vi "Restore Connection.vi"(8 "error in (no error)":errorcluster, 11 "Spectrum Recorder too in":refnum<class "Spectrum Recorder too.lvclass">) -> (0 "error out":errorcluster, 1 "Attempts":i32, 2 "Time elapsed, ms":u32, 3 "Spectrum Recorder too out":refnum<class "Spectrum Recorder too.lvclass">)   [LabVIEW 2020, in "Spectrum Recorder too.lvclass"]
uses:
  Spectrum Recorder too.lvclass
  <vilib>/Utility/error.llb/Error Cluster From Error Code.vi
  <vilib>/ErrorRing/Error Ring.xnode
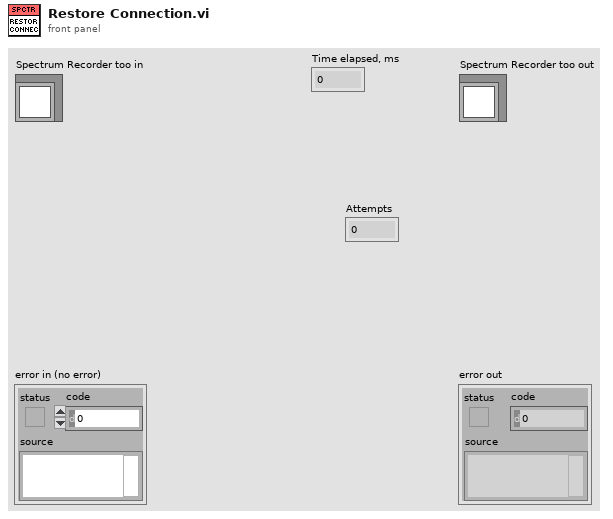
[diagram p1: front panel]
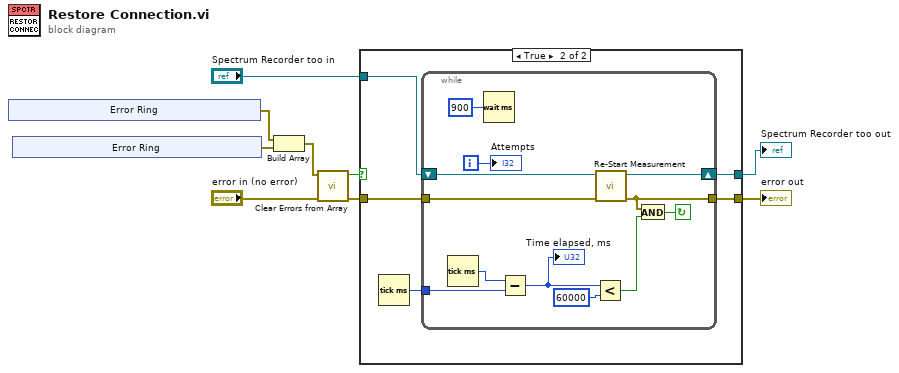
[diagram p0: block diagram]
diagram:
  n1 = xnode "Error Ring"() -> ("error out"=w9:errorcluster)
  n2 = xnode "Error Ring"() -> ("error out"=w8:errorcluster)
  n3 = Build Array(w9, w8) -> (w7:errorcluster[])
  n4 = call "Clear Errors from Array.vi"("Error In"="error in (no error)", "Errors to clear"=w7) -> ("Error Out"=w5:errorcluster, "specific error cleared?"=w6:bool)  [unwired: 8 in]
  n5 = case shown="True" w6 {
    tunnel: w5 -> [w11 w14]
    tunnel: "Spectrum Recorder too in" -> [w10 w15]
    tunnel: [w11 w13] -> w3
    tunnel: [w10 w12] -> w1
    frame False {
    }
    frame True {
      n6 = Tick Count (ms)() -> (millisecond timer value=w16:u32)
      n7 = while {
        tunnel: w16 -> [w25]
        tunnel: w14 -> [w27]
        tunnel: [w18] -> w13
        shift-right: [w21] -> w12
        shift-left: w15 -> [w28]
        i -> [w19]
        stop <- w22 continue-if-true
        n8 = Tick Count (ms)() -> (millisecond timer value=w26:u32)
        n9 = Wait (ms)(milliseconds to wait=u32 900) -> ()  [unwired: 1 out]
        n10 = Subtract(x=w26, y=w25) -> (x-y=w24:u32)
        "Time elapsed, ms" <- w24
        n11 = Less?(x=w24, y=60000) -> (x < y?=w17:bool)
        n12 = call-dynamic "Re-Start Measurement.vi"("error in (no error)"=w27, "Spectrum Recorder too in"=w28) -> ("error out"=w18:errorcluster, "Spectrum Recorder too out"=w21:refnum<class "Spectrum Recorder too.lvclass">)  [unwired: 8 in]
        n13 = And(x=w18, y=w17) -> (x .and. y?=w22:bool)
        "Attempts" <- w19
      }
    }
  }
  "error out" <- w3
  "Spectrum Recorder too out" <- w1
